vi "measureCombs_anySet.vi"(3 "Read freqs. \nfrom textfile":bool, 5 "Cluster":T2={"span"=300000000.0, "rbw"=10000.0, "enableVBW"=FALSE, "vbw"=0.0, "traceLength"=64001, "window"=0, "verticalUnit"=0, "center freq"=150000000.0} {"verticalUnit" items=["SpectrumVerticalUnit_dBm", "SpectrumVerticalUnit_Watt", "SpectrumVerticalUnit_Volt", "SpectrumVerticalUnit_Amp", "SpectrumVerticalUnit_dBmV"]; "window" items=["SpectrumWindow_Kaiser", "SpectrumWindow_Mil6dB", "SpectrumWindow_BlackmanHarris", "SpectrumWindow_Rectangle", "SpectrumWindow_FlatTop", "SpectrumWindow_Hann"]; "traceLength" items=["801"=801, "2401"=2401, "4001"=4001, "8001"=8001, "10401"=10401, "16001"=16001, "32001"=32001, "64001"=64001]}, 6 "error in":errorcluster, 7 "Burn time/ RFC measurement time":i32=2, 8 "AFC & OFC Measurement time":i32=2, 9 "Folder for all data (Don't forget the last slash!)":string="C:\\Users\\Lab\\Desktop\\Data\\2019-08\\2019-08-07\\") -> (0 "error out":errorcluster)   [LabVIEW 2016]
uses:
  <vilib>/Utility/file.llb/Read Delimited Spreadsheet (DBL).vi
  <vilib>/Utility/file.llb/Write Delimited Spreadsheet (DBL).vi
panel:
  out "To change these settings, you must edit them in the block diagram":T1(array[cluster])
  in  "Sweep probe twice":bool
  out "Current set #":i32
  out "Current freq.":dbl
  in  "freqs. file":path
  in  "Shuffle?":bool
  in  "Start freq":dbl=1000000.0 format="%0.2e"
  in  "End freq":dbl=2000000.0 format="%0.2e"
  in  "Freq step":i32=100000 format="%.2e"
  out "Duration array":T3(array[cluster])
  in  "Mod shape":enum16{"Triangle", "Sine"}(ring)
  # "consecutive sweeps can be compared\nto check for probe on AFC."
  # "RSA settings"
  # "Suppose you want to collect comb data, first ascending, then descending.\n\nIn Matlab, create a 1xM array \ncontaining all modulation freqs (Hz) in the ascending sequence; then create a 1xN array for the descending case. Note that M != N is fine.\n\nfid= fopen(FILENAME, 'w');\nfprintf(fid,'%d\\t', ARRAY1);\nfprintf(fid,'\\r\\n');\nfprintf(fid,'%d\\t',ARRAY2);\n... \n(for more sets, repeat as needed)\nfclose(fid);\n\nNow find the file you just made:"
  # "Modulation settings"
  # "(zero-indexed)"
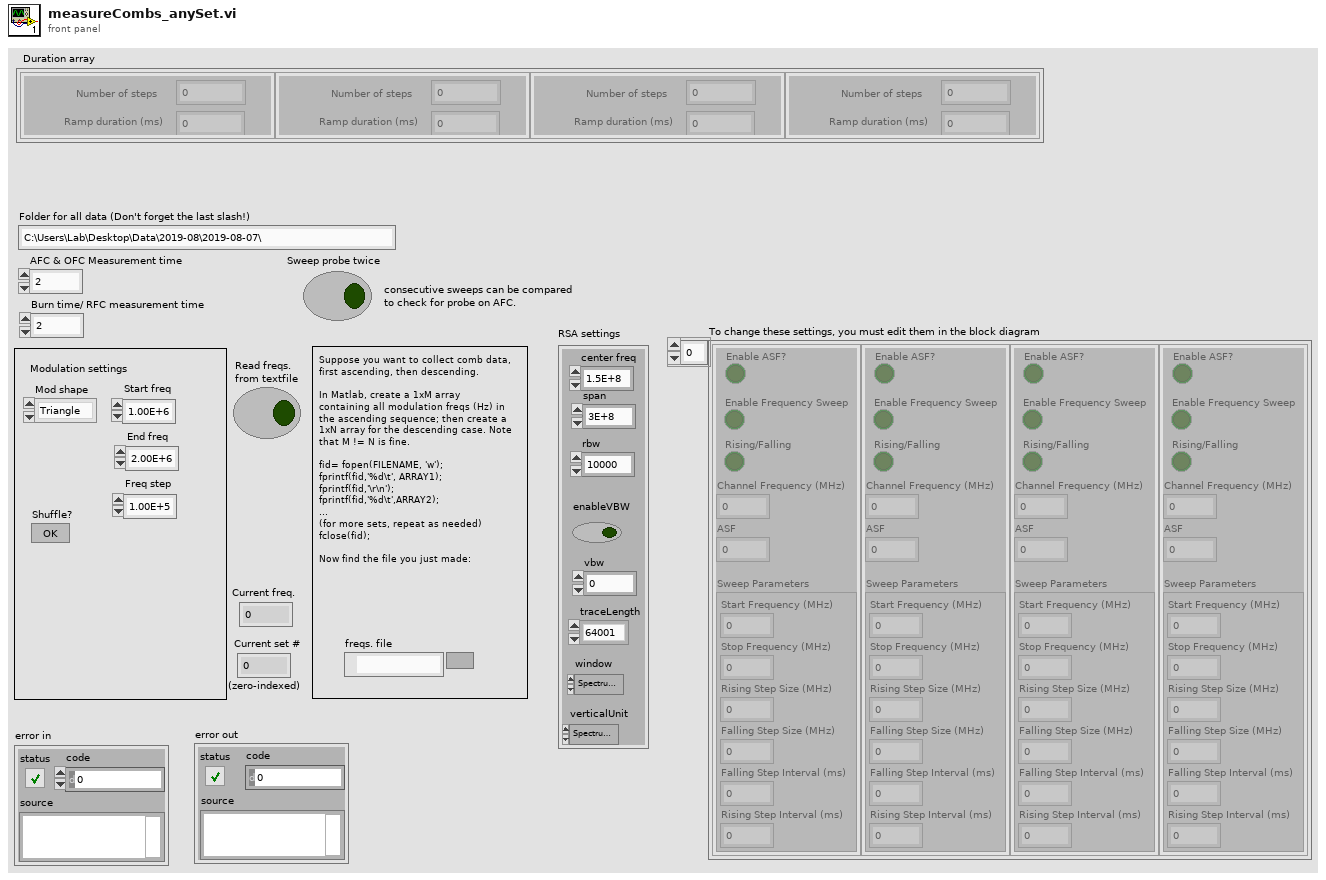
[diagram p1: front panel]
types:
  T1 = cluster{"Enable ASF?":bool, "Channel Frequency (MHz)":dbl, "ASF":dbl, "Enable Frequency Sweep":bool, "Sweep Parameters":cluster{"Start Frequency (MHz)":dbl, "Stop Frequency (MHz)":dbl, "Rising Step Size (MHz)":dbl, "Falling Step Size (MHz)":dbl, "Falling Step Interval (ms)":dbl, "Rising Step Interval (ms)":dbl}, "Rising/Falling":bool}[]
  T2 = cluster{"span":dbl, "rbw":dbl, "enableVBW":bool, "vbw":dbl, "traceLength":u16, "window":u32, "verticalUnit":u32, "center freq":dbl}
  T3 = cluster{"Number of steps":dbl, "Ramp duration (ms)":dbl}[]
  T4 = cluster{"span":dbl, "rbw":dbl, "enableVBW":bool, "vbw":dbl, "traceLength":u16, "window":u32, "verticalUnit":u32}
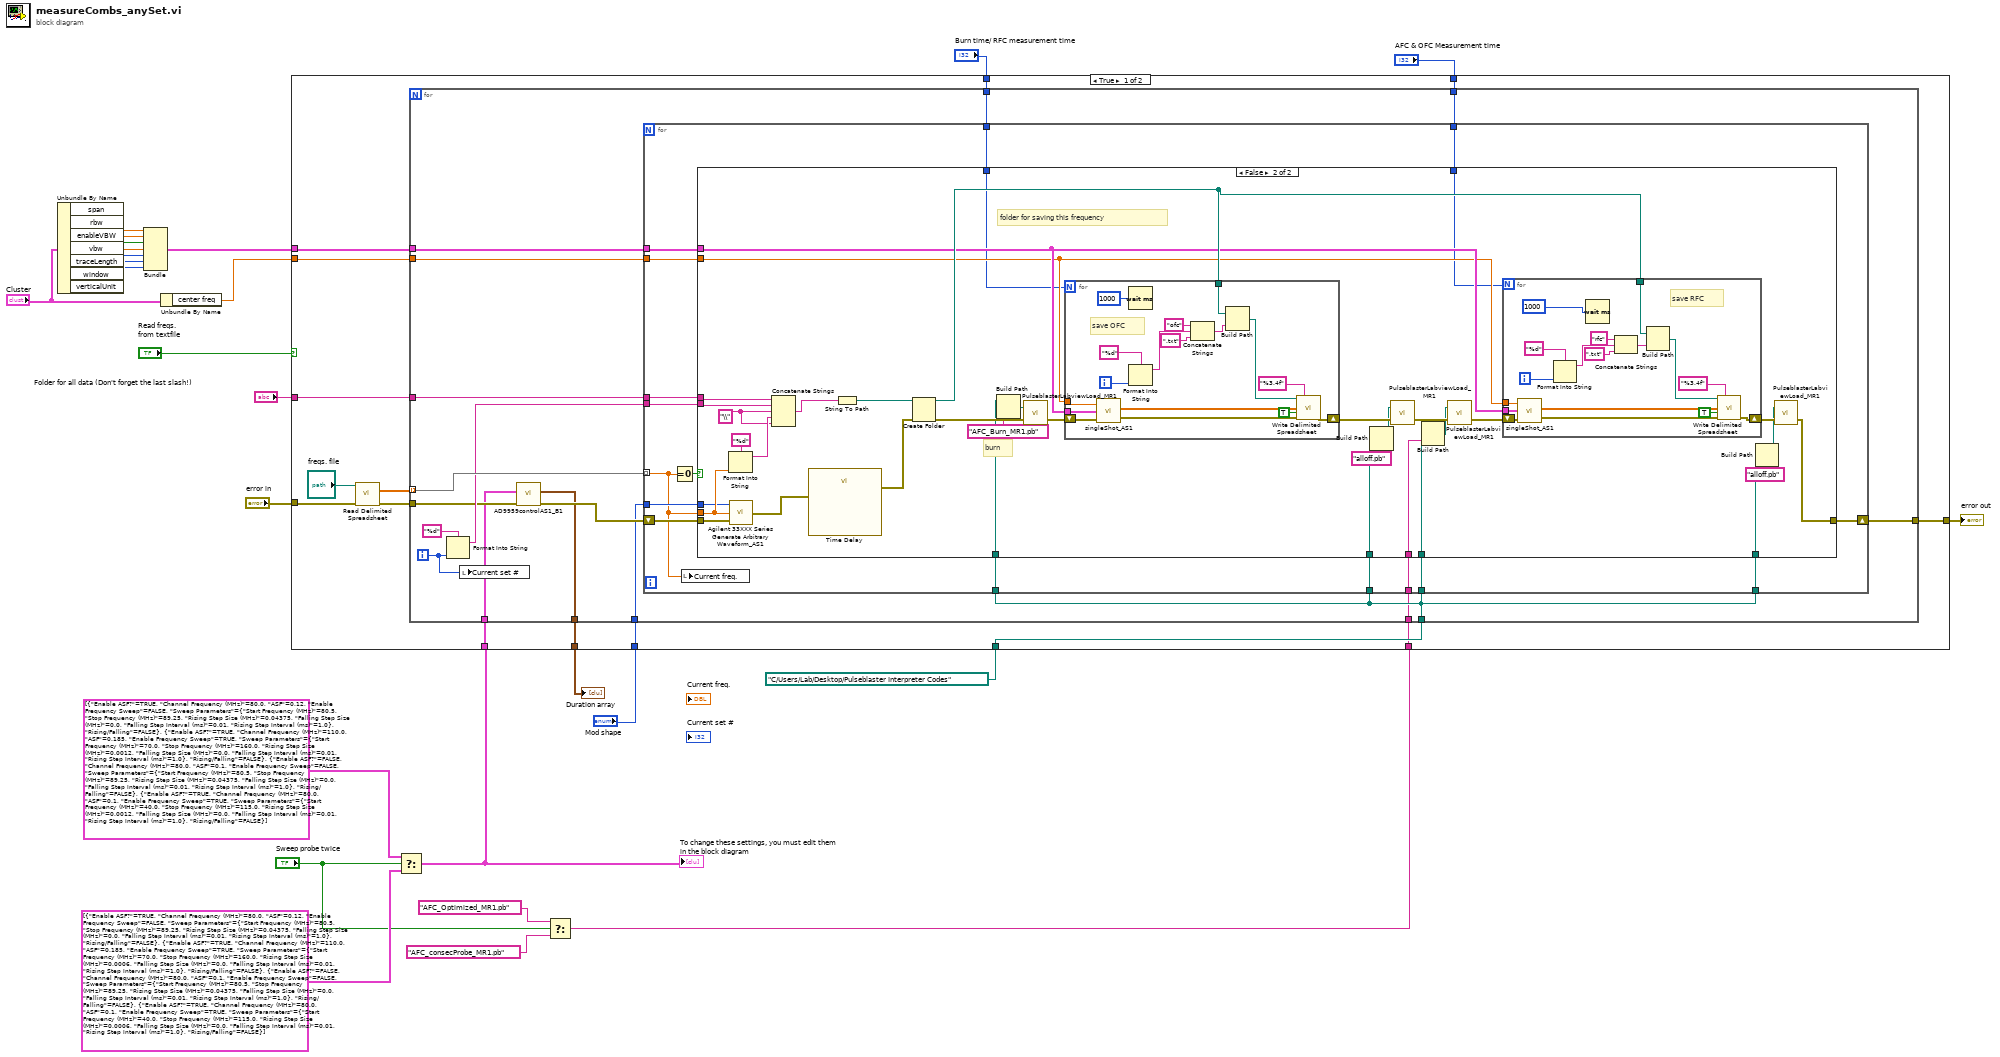
[diagram p0: block diagram]
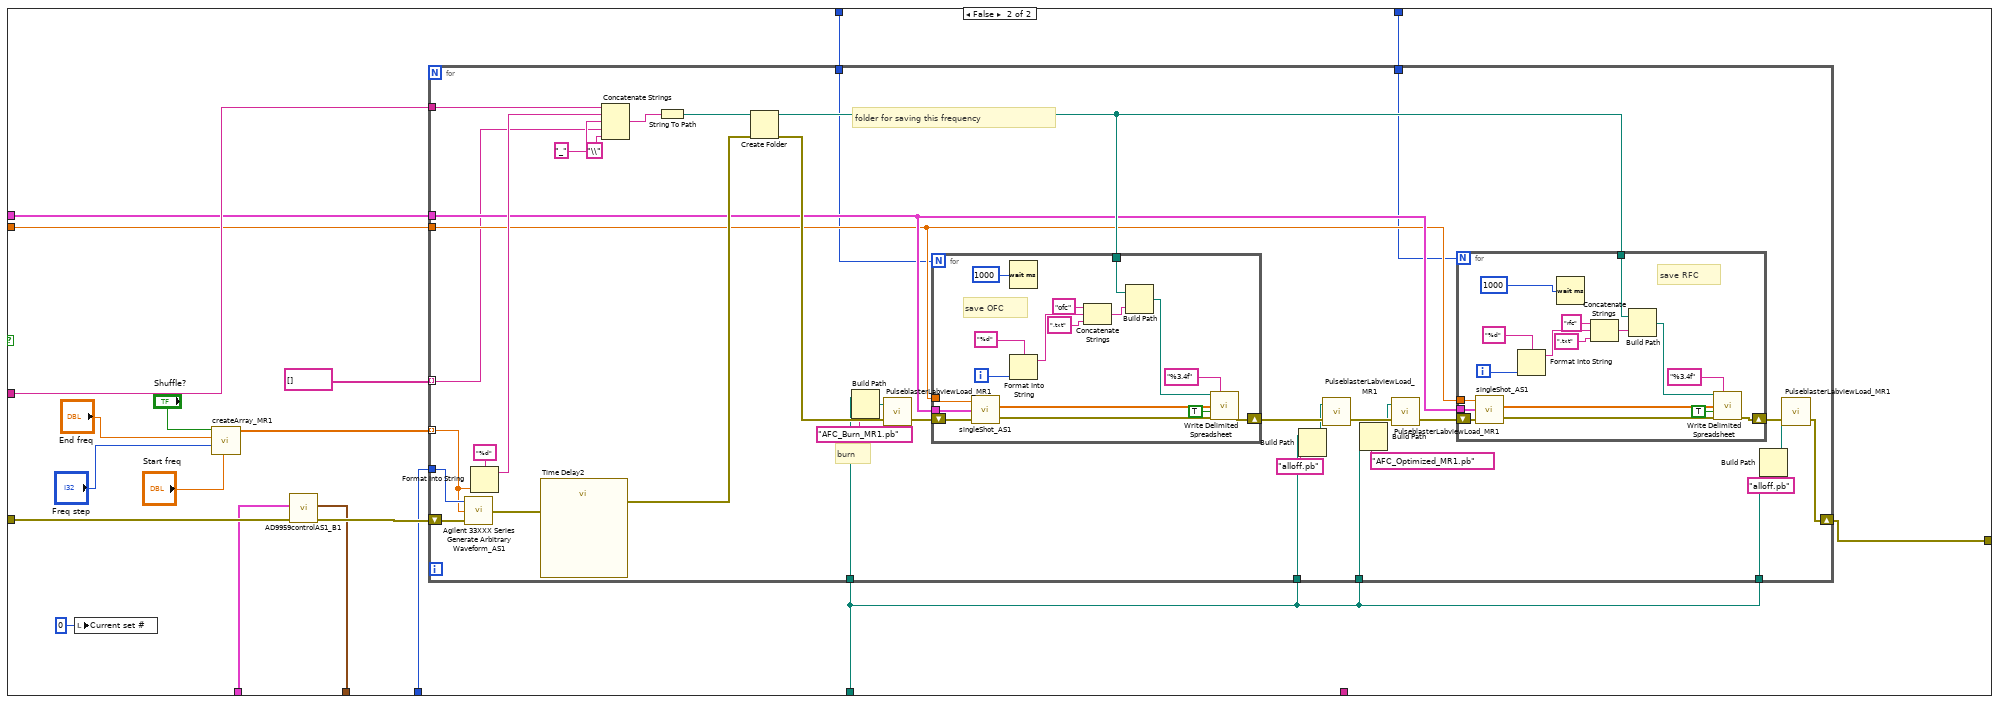
[diagram p3: hidden frame]
diagram:
  n1 = Unbundle By Name("Cluster") -> ("span"=w21:dbl, "rbw"=w20:dbl, "enableVBW"=w19:bool, "vbw"=w18:dbl, "traceLength"=w17:u16, "window"=w16:u32, "verticalUnit"=w15:u32)
  n2 = Bundle("span"=w21, "rbw"=w20, "enableVBW"=w19, "vbw"=w18, "traceLength"=w17, "window"=w16, "verticalUnit"=w15) -> (w14:T4)  [unwired: 1 in]
  n3 = Unbundle By Name("Cluster") -> ("center freq"=w23:dbl)
  n4 = Select(t=T1 [{"Enable ASF?"=TRUE, "Channel Frequency (MHz)"=80.0, "ASF"=0.12, "Enable Frequency Sweep"=FALSE, "Sweep Parameters"={"Start Frequency (MHz)"=80.5, "Stop Frequency (MHz)"=89.25, "Rising Step Size (MHz)"=0.04375, "Falling Step Size (MHz)"=0.0, "Falling Step Interval (ms)"=0.01, "Rising Step Interval (ms)"=1.0}, "Rising/Falling"=FALSE}, {"Enable ASF?"=TRUE, "Channel Frequency (MHz)"=110.0, "ASF"=0.185, "Enable Frequency Sweep"=TRUE, "Sweep Parameters"={"Start Frequency (MHz)"=70.0, "Stop Frequency (MHz)"=160.0, "Rising Step Size (MHz)"=0.0012, "Falling Step Size (MHz)"=0.0, "Falling Step Interval (ms)"=0.01, "Rising Step Interval (ms)"=1.0}, "Rising/Falling"=FALSE}, {"Enable ASF?"=FALSE, "Channel Frequency (MHz)"=80.0, "ASF"=0.1, "Enable Frequency Sweep"=FALSE, "Sweep Parameters"={"Start Frequency (MHz)"=80.5, "Stop Frequency (MHz)"=89.25, "Rising Step Size (MHz)"=0.04375, "Falling Step Size (MHz)"=0.0, "Falling Step Interval (ms)"=0.01, "Rising Step Interval (ms)"=1.0}, "Rising/Falling"=FALSE}, {"Enable ASF?"=TRUE, "Channel Frequency (MHz)"=80.0, "ASF"=0.1, "Enable Frequency Sweep"=TRUE, "Sweep Parameters"={"Start Frequency (MHz)"=40.0, "Stop Frequency (MHz)"=115.0, "Rising Step Size (MHz)"=0.0012, "Falling Step Size (MHz)"=0.0, "Falling Step Interval (ms)"=0.01, "Rising Step Interval (ms)"=1.0}, "Rising/Falling"=FALSE}] ("Array"), s="Sweep probe twice", f=T1 [{"Enable ASF?"=TRUE, "Channel Frequency (MHz)"=80.0, "ASF"=0.12, "Enable Frequency Sweep"=FALSE, "Sweep Parameters"={"Start Frequency (MHz)"=80.5, "Stop Frequency (MHz)"=89.25, "Rising Step Size (MHz)"=0.04375, "Falling Step Size (MHz)"=0.0, "Falling Step Interval (ms)"=0.01, "Rising Step Interval (ms)"=1.0}, "Rising/Falling"=FALSE}, {"Enable ASF?"=TRUE, "Channel Frequency (MHz)"=110.0, "ASF"=0.185, "Enable Frequency Sweep"=TRUE, "Sweep Parameters"={"Start Frequency (MHz)"=70.0, "Stop Frequency (MHz)"=160.0, "Rising Step Size (MHz)"=0.0006, "Falling Step Size (MHz)"=0.0, "Falling Step Interval (ms)"=0.01, "Rising Step Interval (ms)"=1.0}, "Rising/Falling"=FALSE}, {"Enable ASF?"=FALSE, "Channel Frequency (MHz)"=80.0, "ASF"=0.1, "Enable Frequency Sweep"=FALSE, "Sweep Parameters"={"Start Frequency (MHz)"=80.5, "Stop Frequency (MHz)"=89.25, "Rising Step Size (MHz)"=0.04375, "Falling Step Size (MHz)"=0.0, "Falling Step Interval (ms)"=0.01, "Rising Step Interval (ms)"=1.0}, "Rising/Falling"=FALSE}, {"Enable ASF?"=TRUE, "Channel Frequency (MHz)"=80.0, "ASF"=0.1, "Enable Frequency Sweep"=TRUE, "Sweep Parameters"={"Start Frequency (MHz)"=40.0, "Stop Frequency (MHz)"=115.0, "Rising Step Size (MHz)"=0.0006, "Falling Step Size (MHz)"=0.0, "Falling Step Interval (ms)"=0.01, "Rising Step Interval (ms)"=1.0}, "Rising/Falling"=FALSE}] ("Array")) -> (s? t:f=w5:T1)
  "To change these settings, you must edit them in the block diagram" <- w5
  n5 = Select(t="AFC_Optimized_MR1.pb" ("name or relative path"), s="Sweep probe twice", f="AFC_consecProbe_MR1.pb" ("name or relative path")) -> (s? t:f=w1:string)
  n6 = case shown="True" "Read freqs. \nfrom textfile" {
    tunnel: [w41 w164] -> w26
    tunnel: "Folder for all data (Don't forget the last slash!)" -> [w40 w163]
    tunnel: path "C:/Users/Lab/Desktop/Pulseblaster Interpreter Codes" ("base path") -> [w28 w162]
    tunnel: w23 -> [w39 w160]
    tunnel: w14 -> [w38 w159]
    tunnel: "Burn time/ RFC measurement time" -> [w37 w158]
    tunnel: "AFC & OFC Measurement time" -> [w36 w157]
    tunnel: "error in" -> [w34 w150]
    tunnel: "Mod shape" -> [w31 w149]
    tunnel: w5 -> [w30 w148]
    tunnel: [w29 w147] -> w8
    tunnel: w1 -> [w27 _]
    frame True {
      n7 = call-poly <vilib>:"Read Delimited Spreadsheet.vi"("file path (dialog if empty)"="freqs. file", "error in (no error)"=w34) -> ("all rows"=w33:dbl[][], "error out"=w32:errorcluster)  [unwired: 8 in, 4 out]
      n8 = for {
        tunnel: [w58] -> w41
        tunnel: w40 -> [w57]
        tunnel: w28 -> [w56]
        tunnel: w39 -> [w54]
        tunnel: w38 -> [w53]
        tunnel: w37 -> [w52]
        tunnel: w36 -> [w51]
        tunnel: w33 -> [w50] mode=indexing
        tunnel: w32 -> [w47]
        tunnel: w31 -> [w46]
        tunnel: w30 -> [w45]
        tunnel: [w44] -> w29
        tunnel: w27 -> [w42]
        i -> [w43]
        n9 = Format Into String(format string="%d", w43) -> (resulting string=w48:string)  [unwired: 2 in, 1 out]
        n10 = local write "Current set #"(w43) -> ()
        n11 = call "AD9959controlAS1_B1.vi"("error in (no error)"=w47, "Array"=w45) -> ("error out 2"=w55:errorcluster, "Duration array"=w44:T3)  [unwired: 8 in]
        n12 = for {
          tunnel: w50 -> [w60] mode=indexing
          tunnel: w46 -> [w74]
          shift-right: [w73] -> w58
          shift-left: w55 -> [w72]
          tunnel: w57 -> [w62]
          tunnel: w53 -> [w67]
          tunnel: w56 -> [w71]
          tunnel: w56 -> [w70]
          tunnel: w56 -> [w69]
          tunnel: w56 -> [w68]
          tunnel: w54 -> [w66]
          tunnel: w52 -> [w65]
          tunnel: w51 -> [w64]
          tunnel: w48 -> [w63]
          tunnel: w42 -> [w59]
          n13 = Equal To 0?(x=w60) -> (x = 0?=w61:bool)
          n14 = local write "Current freq."(w60) -> ()
          n15 = case shown="False" w61 {
            tunnel: w74 -> [_ w77]
            tunnel: [w75 w111] -> w73
            tunnel: w72 -> [w75 w79]
            tunnel: w71 -> [_ w100]
            tunnel: w70 -> [_ w97]
            tunnel: w69 -> [_ w95]
            tunnel: w68 -> [_ w92]
            tunnel: w67 -> [_ w90]
            tunnel: w66 -> [_ w89]
            tunnel: w65 -> [_ w88]
            tunnel: w64 -> [_ w87]
            tunnel: w63 -> [_ w82]
            tunnel: w62 -> [_ w83]
            tunnel: w60 -> [_ w78]
            tunnel: w59 -> [_ w76]
            frame True {
            }
            frame False {
              w85 = "\\" ("string")
              # "folder for saving this frequency"
              # "burn"
              n16 = Format Into String(format string="%d", w78) -> (resulting string=w86:string)  [unwired: 2 in, 1 out]
              n17 = call "Agilent 33XXX Series Generate Arbitrary Waveform_AS1.vi"("error in (no error)"=w79, "Frequency (1000 Hz)"=w78, "Enum"=w77) -> ("error out"=w80:errorcluster)
              n18 = Concatenate Strings(w83, w82, w85, w86, w85) -> (w81:string)
              n19 = call "Time Delay"("error in (no error)"=w80) -> ("error out"=w104:errorcluster)  [unwired: 10 in]
              n20 = String To Path(string=w81) -> (path=w101:path)
              n21 = Create Folder(path (use dialog)=w101, error in=w104) -> (created path=w102:path, error out=w103:errorcluster)  [unwired: 1 in, 1 out]
              n22 = Build Path(base path=w100, name or relative path="AFC_Burn_MR1.pb") -> (appended path=w98:path)
              n23 = call "PulseblasterLabviewLoad_MR1.vi"("error in (no error)"=w103, "Input file"=w98) -> ("error out"=w110:errorcluster)  [unwired: 1 out]
              n24 = for {
                N: w88 -> [_]
                shift-right: [w142] -> w105
                shift-left: w110 -> [w145]
                tunnel: w102 -> [w133]
                tunnel: w90 -> [w129]
                tunnel: w89 -> [w130]
                i -> [w131]
                # "save OFC"
                n25 = call "singleShot_AS1.vi"("error in"=w145, "Cluster"=w129, "center freq"=w130) -> ("error out"=w144:errorcluster, "traceData out"=w141:sgl[])
                n26 = Wait (ms)(milliseconds to wait=u32 1000) -> ()  [unwired: 1 out]
                n27 = Format Into String(format string="%d", w131) -> (resulting string=w137:string)  [unwired: 2 in, 1 out]
                n28 = Concatenate Strings("ofc" ("string"), w137, ".txt" ("string")) -> (w136:string)
                n29 = Build Path(base path=w133, name or relative path=w136) -> (appended path=w140:path)
                n30 = call-poly <vilib>:"Write Delimited Spreadsheet.vi"("file path (dialog if empty)"=w140, "format (%.3f)"="%3.4f", "1D data"=w141, "append to file? (new file:F)"=TRUE, "error in (no error)"=w144) -> ("error out"=w142:errorcluster)  [unwired: 9 in, 1 out]
              }
              n31 = Build Path(base path=w95, name or relative path="alloff.pb") -> (appended path=w94:path)
              n32 = call "PulseblasterLabviewLoad_MR1.vi"("error in (no error)"=w105, "Input file"=w94) -> ("error out"=w106:errorcluster)  [unwired: 1 out]
              n33 = Build Path(base path=w97, name or relative path=w76) -> (appended path=w96:path)
              n34 = call "PulseblasterLabviewLoad_MR1.vi"("error in (no error)"=w106, "Input file"=w96) -> ("error out"=w108:errorcluster)  [unwired: 1 out]
              n35 = for {
                N: w87 -> [_]
                shift-right: [w125] -> w107
                shift-left: w108 -> [w128]
                tunnel: w90 -> [w112]
                tunnel: w102 -> [w115]
                tunnel: w89 -> [w113]
                i -> [w120]
                # "save RFC"
                n36 = call "singleShot_AS1.vi"("error in"=w128, "Cluster"=w112, "center freq"=w113) -> ("error out"=w127:errorcluster, "traceData out"=w124:sgl[])
                n37 = Format Into String(format string="%d", w120) -> (resulting string=w119:string)  [unwired: 2 in, 1 out]
                n38 = Wait (ms)(milliseconds to wait=u32 1000) -> ()  [unwired: 1 out]
                n39 = Concatenate Strings("rfc" ("string"), w119, ".txt" ("string")) -> (w118:string)
                n40 = Build Path(base path=w115, name or relative path=w118) -> (appended path=w123:path)
                n41 = call-poly <vilib>:"Write Delimited Spreadsheet.vi"("file path (dialog if empty)"=w123, "format (%.3f)"="%3.4f", "1D data"=w124, "append to file? (new file:F)"=TRUE, "error in (no error)"=w127) -> ("error out"=w125:errorcluster)  [unwired: 9 in, 1 out]
              }
              n42 = Build Path(base path=w92, name or relative path="alloff.pb") -> (appended path=w91:path)
              n43 = call "PulseblasterLabviewLoad_MR1.vi"("error in (no error)"=w107, "Input file"=w91) -> ("error out"=w111:errorcluster)  [unwired: 1 out]
            }
          }
        }
      }
    }
    frame False {
      n44 = local write "Current set #"(0 ("Current set #")) -> ()
      n45 = call "createArray_MR1.vi"("Start freq"="Start freq", "Freq step"="Freq step", "End freq"="End freq", "Shuffle?"="Shuffle?") -> ("Riffled {X}"=w151:dbl[])  [unwired: 7 in]
      n46 = call "AD9959controlAS1_B1.vi"("error in (no error)"=w150, "Array"=w148) -> ("error out 2"=w161:errorcluster, "Duration array"=w147:T3)  [unwired: 8 in]
      n47 = for {
        tunnel: w151 -> [w165] mode=indexing
        tunnel: w149 -> [w201]
        shift-right: [w200] -> w164
        shift-left: w161 -> [w199]
        tunnel: w163 -> [w173]
        tunnel: w159 -> [w172]
        tunnel: w162 -> [w184]
        tunnel: w162 -> [w181]
        tunnel: w162 -> [w178]
        tunnel: w162 -> [w175]
        tunnel: w160 -> [w171]
        tunnel: w158 -> [w170]
        tunnel: w157 -> [w169]
        tunnel: string[] [] -> [w166] mode=indexing
        # "folder for saving this frequency"
        # "burn"
        n48 = call "Agilent 33XXX Series Generate Arbitrary Waveform_AS1.vi"("error in (no error)"=w199, "Frequency (1000 Hz)"=w165, "Enum"=w201) -> ("error out"=w194:errorcluster)
        n49 = Format Into String(format string="%d", w165) -> (resulting string=w196:string)  [unwired: 2 in, 1 out]
        n50 = call "Time Delay2"("error in (no error)"=w194) -> ("error out"=w189:errorcluster)  [unwired: 10 in]
        n51 = Concatenate Strings(w173, w196, "_" ("string"), w166, "\\" ("string")) -> (w186:string)
        n52 = String To Path(string=w186) -> (path=w185:path)
        n53 = Create Folder(path (use dialog)=w185, error in=w189) -> (created path=w187:path, error out=w188:errorcluster)  [unwired: 1 in, 1 out]
        n54 = Build Path(base path=w184, name or relative path="AFC_Burn_MR1.pb") -> (appended path=w182:path)
        n55 = call "PulseblasterLabviewLoad_MR1.vi"("error in (no error)"=w188, "Input file"=w182) -> ("error out"=w198:errorcluster)  [unwired: 1 out]
        n56 = for {
          N: w170 -> [_]
          shift-right: [w232] -> w190
          shift-left: w198 -> [w235]
          tunnel: w187 -> [w223]
          tunnel: w172 -> [w219]
          tunnel: w171 -> [w220]
          i -> [w221]
          # "save OFC"
          n57 = call "singleShot_AS1.vi"("error in"=w235, "Cluster"=w219, "center freq"=w220) -> ("error out"=w234:errorcluster, "traceData out"=w231:sgl[])
          n58 = Wait (ms)(milliseconds to wait=u32 1000) -> ()  [unwired: 1 out]
          n59 = Format Into String(format string="%d", w221) -> (resulting string=w227:string)  [unwired: 2 in, 1 out]
          n60 = Concatenate Strings("ofc" ("string"), w227, ".txt" ("string")) -> (w226:string)
          n61 = Build Path(base path=w223, name or relative path=w226) -> (appended path=w230:path)
          n62 = call-poly <vilib>:"Write Delimited Spreadsheet.vi"("file path (dialog if empty)"=w230, "format (%.3f)"="%3.4f", "1D data"=w231, "append to file? (new file:F)"=TRUE, "error in (no error)"=w234) -> ("error out"=w232:errorcluster)  [unwired: 9 in, 1 out]
        }
        n63 = Build Path(base path=w178, name or relative path="alloff.pb") -> (appended path=w177:path)
        n64 = call "PulseblasterLabviewLoad_MR1.vi"("error in (no error)"=w190, "Input file"=w177) -> ("error out"=w191:errorcluster)  [unwired: 1 out]
        n65 = Build Path(base path=w181, name or relative path="AFC_Optimized_MR1.pb") -> (appended path=w179:path)
        n66 = call "PulseblasterLabviewLoad_MR1.vi"("error in (no error)"=w191, "Input file"=w179) -> ("error out"=w193:errorcluster)  [unwired: 1 out]
        n67 = for {
          N: w169 -> [_]
          shift-right: [w215] -> w192
          shift-left: w193 -> [w218]
          tunnel: w172 -> [w202]
          tunnel: w187 -> [w205]
          tunnel: w171 -> [w203]
          i -> [w210]
          # "save RFC"
          n68 = call "singleShot_AS1.vi"("error in"=w218, "Cluster"=w202, "center freq"=w203) -> ("error out"=w217:errorcluster, "traceData out"=w214:sgl[])
          n69 = Format Into String(format string="%d", w210) -> (resulting string=w209:string)  [unwired: 2 in, 1 out]
          n70 = Wait (ms)(milliseconds to wait=u32 1000) -> ()  [unwired: 1 out]
          n71 = Concatenate Strings("rfc" ("string"), w209, ".txt" ("string")) -> (w208:string)
          n72 = Build Path(base path=w205, name or relative path=w208) -> (appended path=w213:path)
          n73 = call-poly <vilib>:"Write Delimited Spreadsheet.vi"("file path (dialog if empty)"=w213, "format (%.3f)"="%3.4f", "1D data"=w214, "append to file? (new file:F)"=TRUE, "error in (no error)"=w217) -> ("error out"=w215:errorcluster)  [unwired: 9 in, 1 out]
        }
        n74 = Build Path(base path=w175, name or relative path="alloff.pb") -> (appended path=w174:path)
        n75 = call "PulseblasterLabviewLoad_MR1.vi"("error in (no error)"=w192, "Input file"=w174) -> ("error out"=w200:errorcluster)  [unwired: 1 out]
      }
    }
  }
  "error out" <- w26
  "Duration array" <- w8
